vi "Read Displacement Derived.vi"(11 "StiffnessMonitor in":refnum<class "StiffnessMonitor.lvclass">) -> (2 "Displacement Derived":dbl[unit]=1.0 min=1.0 max=300.0 format="%.1f", 3 "StiffnessMonitor out":refnum<class "StiffnessMonitor.lvclass">)   [LabVIEW 2013, in "StiffnessMonitor.lvclass"]
uses:
  StiffnessMonitor.lvclass
  StiffnessMonitor.lvclass/StiffnessMonitor.ctl
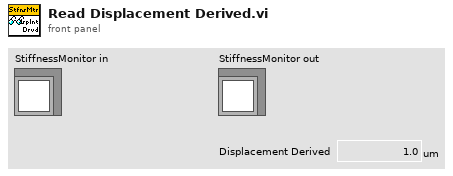
[diagram p1: front panel]
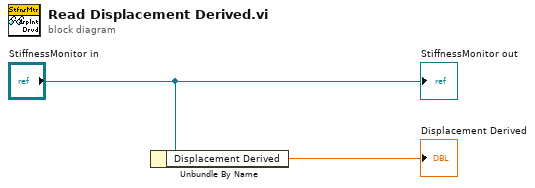
[diagram p0: block diagram]
diagram:
  n1 = Unbundle By Name("StiffnessMonitor in") -> ("Displacement Derived"=→"Displacement Derived":dbl[unit])
  "StiffnessMonitor out" <- "StiffnessMonitor in"
